vi "waitExample.vi"() -> ()   [LabVIEW 2014]
panel:
  out "Clock Ticker \nIndicator":string
  in  "Stop Button \nControl":bool
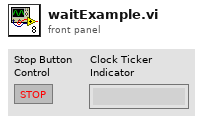
[diagram p1: front panel]
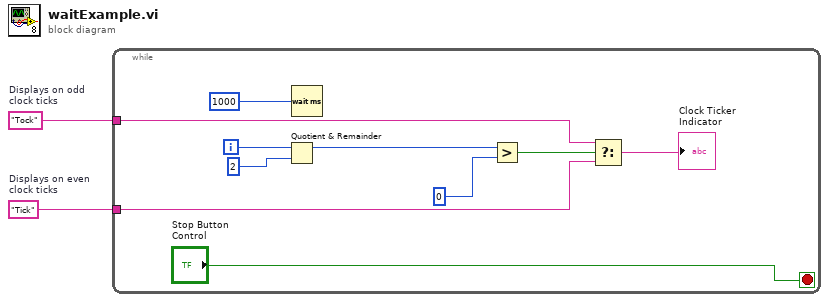
[diagram p0: block diagram]
diagram:
  w2 = "Tick"  # Displays on even clock ticks
  w1 = "Tock"  # Displays on odd  clock ticks
  n1 = while {
    tunnel: w2 -> [w12]
    tunnel: w1 -> [w11]
    i -> [w10]
    stop <- "Stop Button \nControl" stop-if-true
    n2 = Quotient & Remainder(x=w10, y=2) -> (x-y*floor(x/y)=w8:i32)  [unwired: 1 out]
    n3 = Wait (ms)(milliseconds to wait=u32 1000) -> ()  [unwired: 1 out]
    n4 = Greater?(x=w8, y=0) -> (0:w6:bool)
    n5 = Select(t=w11, s=w6, f=w12) -> (s? t:f=→"Clock Ticker \nIndicator":string)
  }
